vi "Encoder for velocity.vi"() -> ()   [LabVIEW 2020]
uses:
  <vilib>/DAQmx/read.llb/DAQmx Read (Counter DBL 1Chan 1Samp).vi
  <vilib>/DAQmx/read.llb/DAQmx Read (Counter U32 1Chan 1Samp).vi
  <vilib>/DAQmx/miscellaneous.llb/DAQmx Fill In Error Info.vi
  Global-velocity.vi
  Global-trigger.vi
  <vilib>/DAQmx/create/channels.llb/DAQmx Create Channel (CI-Count Edges).vi
  <vilib>/ptbypt/NI_PtbyPt.lvlib
  <resource>/objmgr/daqmx.rc
panel:
  out "Waveform Chart for velocity":dbl(graph)
  in  "Edge?":bool
  in  "stop":bool
  out "edge":u32
  in  "error in":errorcluster
  out "frequence":dbl format="%0.2f"
  in  "radius":dbl
  in  "counts per Revolution":dbl=2048.0
  out "velocity":dbl
  out "Waveform Chart 2":dbl[](graph)
  out "largest Velocity":dbl
  in  "sampling point":i32=500
  out "trigger":bool
  in  "Record start value":dbl=100.0
  out "Waveform Chart for frequency":dbl(graph)
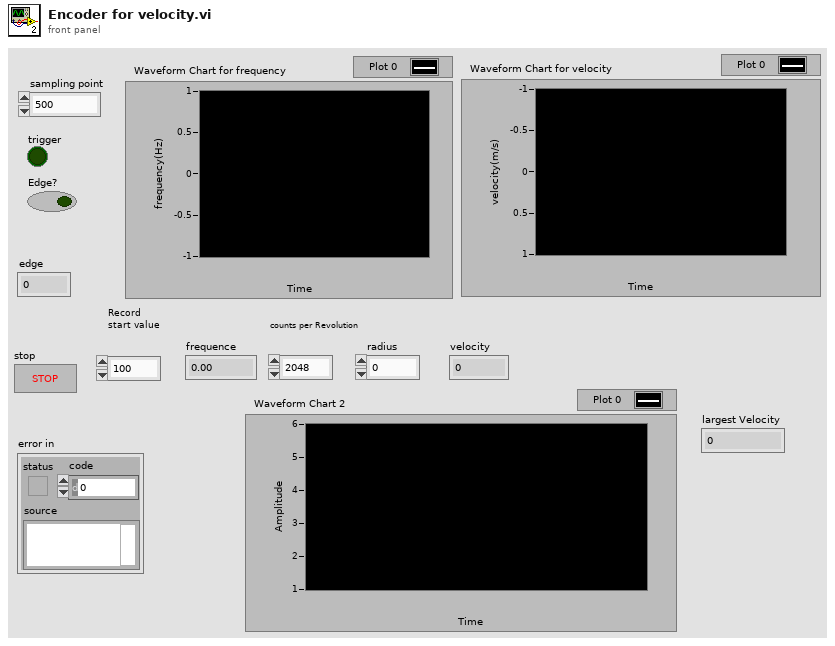
[diagram p1: front panel]
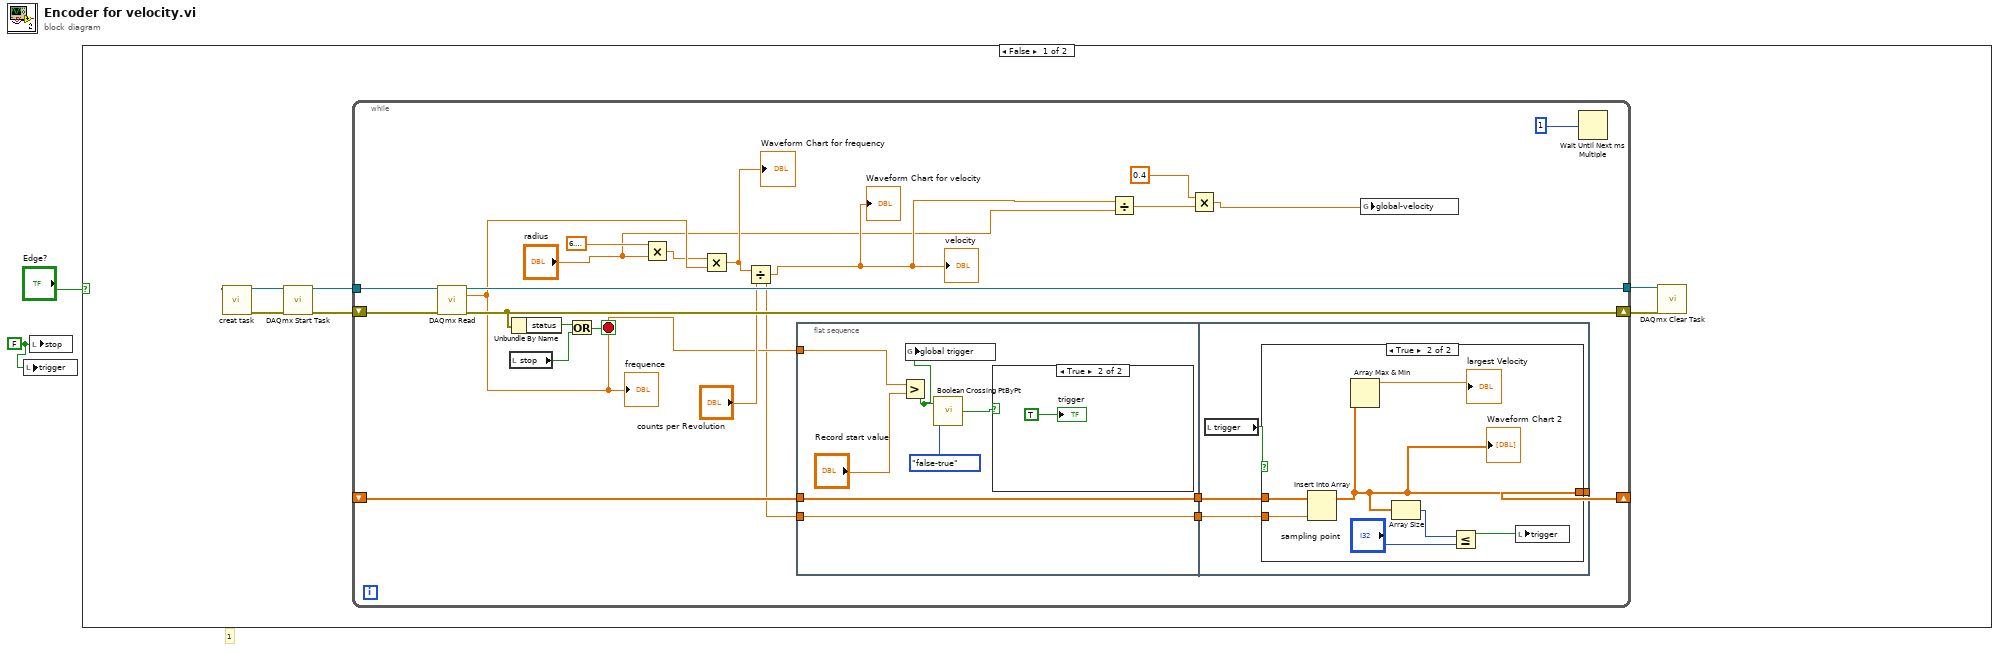
[diagram p0: block diagram]
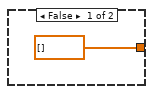
[diagram p3: hidden frame]
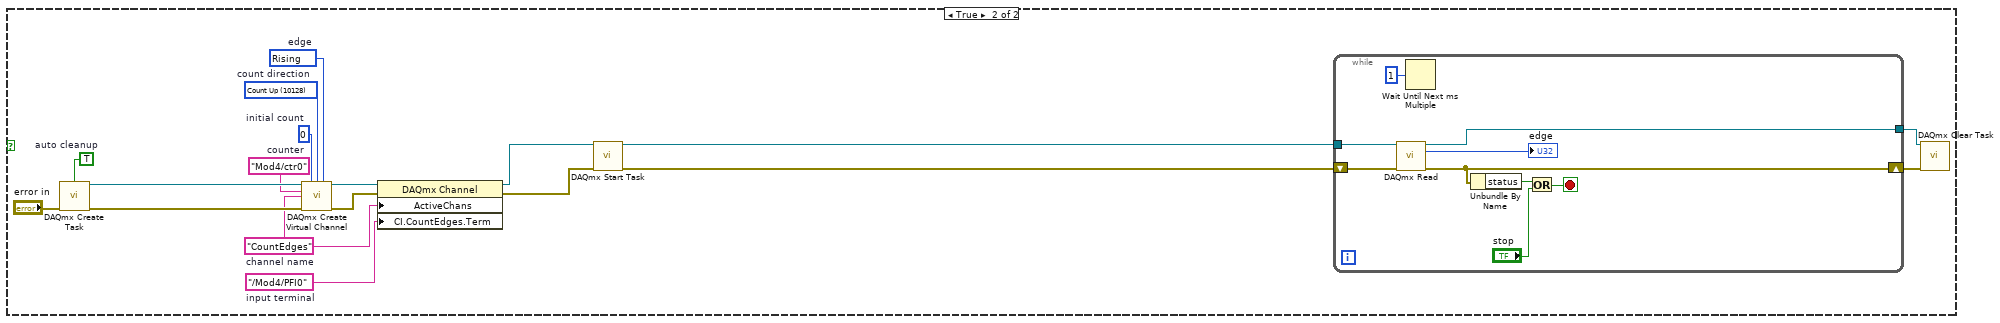
[diagram p4: hidden frame]
diagram:
  w1 = FALSE ("stop")
  # "1"
  n1 = local write "trigger"(w1) -> ()
  n2 = local write "stop"(w1) -> ()
  n3 = case shown="False" "Edge?" {
    frame False {
      n4 = call "creat task.vi"() -> ("error out"=w8:errorcluster, "task out"=w7:refnum<k21>)  [unwired: 10 in]
      n5 = call <vilib>:"DAQmx Start Task.vi"("task/channels in"=w7, "error in"=w8) -> ("task out"=w3:refnum<k21>, "error out"=w4:errorcluster)  [unwired: 12 in]
      n6 = while {
        tunnel: w3 -> [w30]
        tunnel: [w28] -> w6
        shift-right: [w27] -> w5
        shift-left: w4 -> [w29]
        shift-right: [w21] -> _
        shift-left: _ -> [w20]
        stop <- w25 stop-if-true
        n7 = call-poly <vilib>:"DAQmx Read.vi"("task/channels in"=w30, "error in"=w29) -> ("task out"=w28:refnum<k21>, "data"=w17:dbl, "error out"=w27:errorcluster)  [unwired: 11 in]
        "frequence" <- w17
        n8 = local read "stop"() -> (w22:bool)
        n9 = Unbundle By Name(w27) -> ("status"=w26:bool)
        n10 = Or(x=w26, y=w22) -> (x .or. y?=w25:bool)
        n11 = Multiply(x=6.283185307179586, y="radius") -> (x*y=w13:dbl)
        n12 = Multiply(x=w13, y=w17) -> (x*y=w15:dbl)
        "Waveform Chart for frequency" <- w15
        n13 = Divide(x=w15, y="counts per Revolution") -> (x/y=w14:dbl)
        "velocity" <- w14
        "Waveform Chart for velocity" <- w14
        n14 = flat-sequence {
          tunnel: w20 -> [w36]
          tunnel: w14 -> [w37]
          tunnel: [w37] -> w19
          tunnel: [w36] -> w18
          tunnel: w17 -> [w34]
          tunnel: [w41] -> w21
          tunnel: w19 -> [w42]
          tunnel: w18 -> [w40]
          frame #0 {
            n15 = Greater?(x=w34, y="Record start value") -> (0:w31:bool)
            n16 = global write "Global-trigger.vi" "global trigger"(w31) -> ()
            n17 = call <vilib>:"Boolean Crossing PtByPt.vi"("direction"=enum16{"either", "false-true", "true-false"}."false-true", "input"=w31) -> ("crossing"=w32:bool)  [unwired: 1 in]
            n18 = case shown="True" w32 {
              frame False {
              }
              frame True {
                "trigger" <- TRUE ("x >= y?")
              }
            }
          }
          frame #1 {
            n19 = local read "trigger"() -> (w39:bool)
            n20 = case shown="True" w39 {
              tunnel: w42 -> [_ w50]
              tunnel: [dbl[] [] w46] -> w41
              tunnel: w40 -> [_ w49]
              frame False {
              }
              frame True {
                n21 = Insert Into Array(array=w49, new element=w50) -> (w46:dbl[])  [unwired: 1 in]
                "Waveform Chart 2" <- w46
                n22 = Array Max & Min(array=w46) -> (max value=→"largest Velocity":dbl)  [unwired: 3 out]
                n23 = Array Size(array=w46) -> (size(s)=w48:i32)
                n24 = Less Or Equal?(x=w48, y="sampling point") -> (x <= y?=w44:bool)
                n25 = local write "trigger"(w44) -> ()
              }
            }
          }
        }
        n26 = Divide(x=w14, y="radius") -> (x/y=w11:dbl)
        n27 = Multiply(x=0.4, y=w11) -> (x*y=w9:dbl)
        n28 = global write "Global-velocity.vi" "global-velocity"(w9) -> ()
        n29 = Wait Until Next ms Multiple(millisecond multiple=u32 1) -> ()  [unwired: 1 out]
      }
      n30 = call <vilib>:"DAQmx Clear Task.vi"("task in"=w6, "error in"=w5) -> ()  [unwired: 13 in, 1 out]
    }
    frame True {
      w53 = "/Mod4/PFI0"  # input terminal
      w56 = 10280 items=["Rising"=10280, "Falling"=10171]  # edge
      w57 = 10128 items=["Count Up"=10128, "Count Down"=10124, "Externally Controlled"=10326]  # count direction
      w58 = u32 0  # initial count
      w54 = "CountEdges"  # channel name
      w60 = "Mod4/ctr0"  # counter
      w62 = TRUE  # auto cleanup
      n31 = call <vilib>:"DAQmx Create Task.vi"("auto cleanup"=w62, "error in"="error in") -> ("task out"=w61:refnum<k21>, "error out"=w63:errorcluster)  [unwired: 12 in]
      n32 = call-poly <vilib>:"DAQmx Create Virtual Channel.vi"("task in"=w61, "initial count"=w58, "count direction"=w57, "edge"=w56, "counter"=w60, "name to assign"=w54, "error in"=w63) -> ("task out"=w55:refnum<k21>, "error out"=w59:errorcluster)  [unwired: 7 in]
      n33 = property class="DAQmx Channel"(reference=w55, error in=w59, "ActiveChans"=w54, "CI.CountEdges.Term"=w53) -> (reference out=w52:refnum<k21>, error out=w51:errorcluster)
      n34 = call <vilib>:"DAQmx Start Task.vi"("task/channels in"=w52, "error in"=w51) -> ("task out"=w68:refnum<k21>, "error out"=w67:errorcluster)  [unwired: 12 in]
      n35 = while {
        tunnel: w68 -> [w77]
        tunnel: [w75] -> w65
        shift-right: [w73] -> w66
        shift-left: w67 -> [w76]
        stop <- w71 stop-if-true
        n36 = call-poly <vilib>:"DAQmx Read.vi"("task/channels in"=w77, "error in"=w76) -> ("task out"=w75:refnum<k21>, "data"=→"edge":u32, "error out"=w73:errorcluster)  [unwired: 11 in]
        n37 = Wait Until Next ms Multiple(millisecond multiple=u32 1) -> ()  [unwired: 1 out]
        n38 = Unbundle By Name(w73) -> ("status"=w74:bool)
        n39 = Or(x=w74, y="stop") -> (x .or. y?=w71:bool)
      }
      n40 = call <vilib>:"DAQmx Clear Task.vi"("task in"=w65, "error in"=w66) -> ()  [unwired: 13 in, 1 out]
    }
  }
